vi "SGL to boolean.vi"(11 "Number":sgl) -> (2 "Numeric 2":u32, 3 "Numeric":u32)   [LabVIEW 2019]
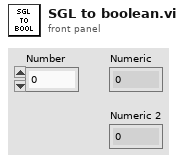
[diagram p1: front panel]
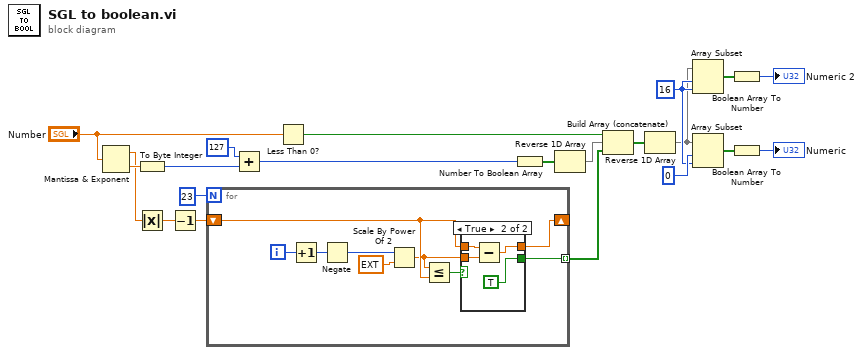
[diagram p0: block diagram]
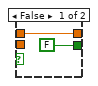
[diagram p2: hidden frame]
diagram:
  w7 = 16 ("length")
  n1 = Mantissa & Exponent(0:"Number") -> (1:w12:sgl, 2:w15:sgl)
  n2 = To Byte Integer(number=w15) -> (8bit integer=w21:i8)
  n3 = Absolute Value(x=w12) -> (abs(x)=w13:sgl)
  n4 = Decrement(x=w13) -> (x-1=w17:sgl)
  n5 = for {
    N: 23 -> [_]
    shift-right: [w23] -> _
    shift-left: w17 -> [w25]
    tunnel: [w22] -> w9 mode=indexing
    i -> [w30]
    n6 = Increment(x=w30) -> (x+1=w29:i32)
    n7 = Negate(x=w29) -> (-x=w28:i32)
    n8 = Scale By Power Of 2(n=w28, x=ext 1.0) -> (x*2^n=w24:ext)
    n9 = Less Or Equal?(x=w24, y=w25) -> (x <= y?=w26:bool)
    n10 = case shown="True" w26 {
      tunnel: w25 -> [w31 w36]
      tunnel: w24 -> [_ w33]
      tunnel: [w31 w35] -> w23
      tunnel: [FALSE TRUE] -> w22
      frame False {
      }
      frame True {
        n11 = Subtract(x=w36, y=w33) -> (x-y=w35:ext)
      }
    }
  }
  n12 = Add(x=i8 127, y=w21) -> (x+y=w20:i8)
  n13 = Less Than 0?(x="Number") -> (x < 0?=w11:bool)
  n14 = Number To Boolean Array(number=w20) -> (Boolean array=w19:bool[])
  n15 = Reverse 1D Array(array=w19) -> (reversed array=w10:bool[])
  n16 = Build Array (concatenate)(w11, w10, w9) -> (w2:bool[])
  n17 = Reverse 1D Array(array=w2) -> (reversed array=w1:bool[])
  n18 = Array Subset(array=w1, index=w7, length=w7) -> (w5:bool[])
  n19 = Array Subset(array=w1, index=0, length=w7) -> (w6:bool[])
  n20 = Boolean Array To Number(Boolean array=w5) -> (number=→"Numeric 2":u32)
  n21 = Boolean Array To Number(Boolean array=w6) -> (number=→"Numeric":u32)
